vi "JSONRPC Server.vi"(6 "LabVIEW Web Service":refnum<class "Web Service.lvclass">) -> ()   [LabVIEW 2016]
uses:
  <vilib>/wsapi/Web Service.lvclass
  <vilib>/NI/NI JSONRPC Server Framework/Classes/Request/Request.lvclass/Request.ctl
  <vilib>/NI/NI JSONRPC Server Framework/Classes/Request/request.Read method.vi
  <vilib>/NI/NI JSONRPC Server Framework/Classes/Request/request.Read params.vi
  <vilib>/NI/NI JSONRPC Server Framework/Classes/params/params.To JSON Tree.vi
  <vilib>/NI/JSON Support for LabVIEW/JSON Value/New JSON Value/New JSON (String).vi
  <vilib>/NI/NI JSONRPC Server Framework/Classes/Server/Add Response (Method Not Found from Request).vi
  <vilib>/NI/NI JSONRPC Server Framework/Classes/Server/Add Response (Result from Request).vi
  <vilib>/NI/NI JSONRPC Server Framework/Classes/Server/Add Response (Server Error from Request).vi
  <vilib>/NI/JSON Support for LabVIEW/JSON Value/JSON Value.lvclass
  <vilib>/NI/NI JSONRPC Server Framework/Classes/Server/JSONRPC Server.lvclass
  <vilib>/NI/NI JSONRPC Server Framework/Classes/Request/Request.lvclass
panel:
  # "Use the web service input terminal to call the VIs on the Service subpalette of the Web Services palette. Do not remove it from the connector pane unless you don't need access to the palette."
  # "Any additional terminals added to the connector pane of a startup VI will be ignored."
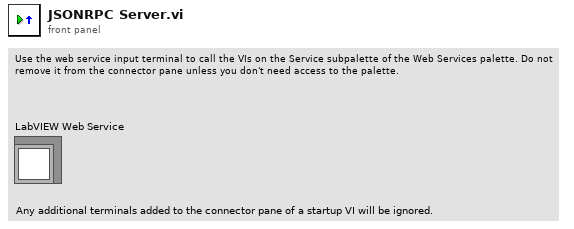
[diagram p1: front panel]
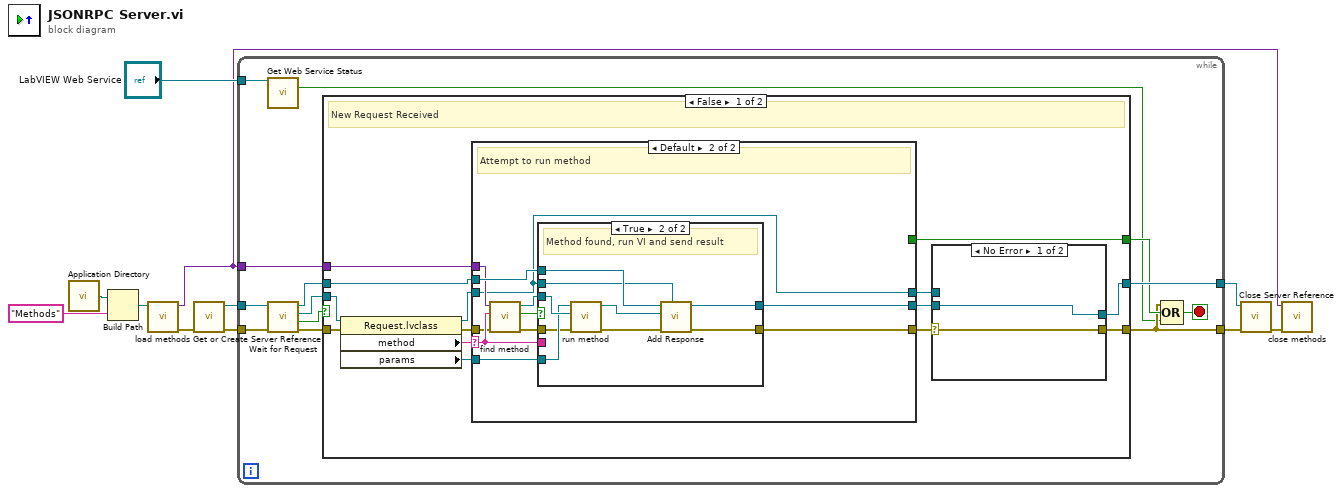
[diagram p0: block diagram]
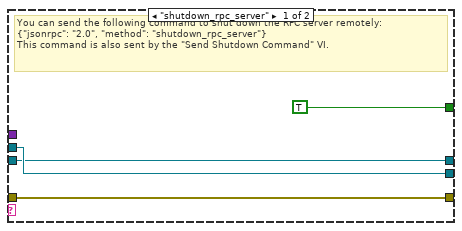
[diagram p2: hidden frame]
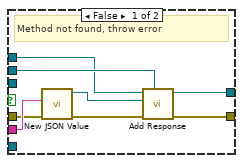
[diagram p3: hidden frame]
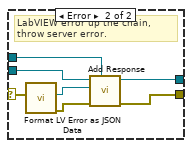
[diagram p4: hidden frame]
diagram:
  n1 = call <vilib>:"Application Directory.vi"() -> ("Application Directory"=w6:path)
  n2 = Build Path(base path=w6, name or relative path="Methods") -> (appended path=w3:path)
  n3 = call "load methods.vi"("Folder Path"=w3) -> ("error out"=w4:errorcluster, "Variant"=w2:variant)  [unwired: 9 in]
  n4 = call <vilib>:"Get or Create Server Reference.vi"("error in (no error)"=w4) -> ("error out"=w10:errorcluster, "Server Out"=w11:refnum<class "JSONRPC Server.lvclass">)  [unwired: 9 in]
  n5 = while {
    tunnel: w11 -> [w24]
    tunnel: w10 -> [w20]
    tunnel: [w16] -> w8
    tunnel: [w18] -> w9
    tunnel: "LabVIEW Web Service" -> [w14]
    tunnel: w2 -> [w12]
    stop <- w15 stop-if-true
    n6 = call <vilib>:"Get Web Service Status.vi"("LabVIEW Web Service"=w14) -> ("service stopping?"=w13:bool)  [unwired: 12 in, 2 out]
    n7 = call <vilib>:"Wait for Request.vi"("error in (no error)"=w20, "Server in"=w24) -> ("error out"=w19:errorcluster, "timed out?"=w21:bool, "Request"=w22:refnum<class "Request.lvclass">, "Server out"=w23:refnum<class "JSONRPC Server.lvclass">)  [unwired: 6 in]
    n8 = case shown="False" w21 {
      tunnel: w23 -> [w29 w80]
      tunnel: w22 -> [w38 _]
      tunnel: w19 -> [w35 w81]
      tunnel: [w30 w81] -> w16
      tunnel: [w33 _] -> w17
      tunnel: [w25 w80] -> w18
      tunnel: w12 -> [w32 _]
      frame False {
        # "New Request Received"
        n9 = property class="Request.lvclass"(reference=w38, error in=w35) -> (reference out=w28:refnum<class "Request.lvclass">, error out=w34:errorcluster, "method"=w37:string, "params"=w36:refnum<class "JSON Value.lvclass">)
        n10 = case shown="Default" w37 {
          selector: w37 -> [_ w49]
          tunnel: w36 -> [_ w50]
          tunnel: w34 -> [w41 w48]
          tunnel: [w41 w52] -> w31
          tunnel: [TRUE _] -> w33
          tunnel: w29 -> [w40 w53]
          tunnel: [w40 w51] -> w26
          tunnel: w28 -> [w39 w43]
          tunnel: w32 -> [_ w44]
          tunnel: [w39 w43] -> w27
          frame "shutdown_rpc_server" {
            # "You can send the following command to shut down the RPC server remotely:\n{\"jsonrpc\": \"2.0\", \"method\": \"shutdown_rpc_server\"}\nThis command is also sent by the \"Send Shutdown Command\" VI."
          }
          frame Default {
            # "Attempt to run method"
            n11 = call "find method.vi"("error in (no error)"=w48, "String"=w49, "Variant"=w44) -> ("error out"=w45:errorcluster, "Boolean"=w46:bool, "VI out"=w47:refnum<vi>)  [unwired: 6 in]
            n12 = case shown="True" w46 {
              tunnel: w53 -> [w60 w70]
              tunnel: w43 -> [w61 w69]
              tunnel: [w58 w68] -> w52
              tunnel: [w59 w67] -> w51
              tunnel: w47 -> [_ w66]
              tunnel: w50 -> [_ w65]
              tunnel: w49 -> [w57 _]
              tunnel: w45 -> [w54 w63]
              frame False {
                # "Method not found, throw error"
                n13 = call-poly <vilib>:"New JSON Value.vi"("error in (no error)"=w54, "value"=w57) -> ("error out"=w55:errorcluster, "JSON Value out"=w56:refnum<class "JSON Value.lvclass">)  [unwired: 8 in]
                n14 = call-poly <vilib>:"Add Response.vi"("Request"=w61, "error in (no error)"=w55, "data"=w56, "Server in"=w60) -> ("error out"=w58:errorcluster, "Server out"=w59:refnum<class "JSONRPC Server.lvclass">)  [unwired: 5 in, 1 out]
              }
              frame True {
                # "Method found, run VI and send result"
                n15 = call "run method.vi"("error in (no error)"=w63, "VI in"=w66, "JSON Value in"=w65) -> ("error out"=w62:errorcluster, "JSON Value out"=w64:refnum<class "JSON Value.lvclass">)  [unwired: 7 in]
                n16 = call-poly <vilib>:"Add Response.vi"("Request"=w69, "error in (no error)"=w62, "JSON Value in"=w64, "Server in"=w70) -> ("error out"=w68:errorcluster, "Server out"=w67:refnum<class "JSONRPC Server.lvclass">)  [unwired: 5 in, 1 out]
              }
            }
          }
        }
        n17 = case shown="No Error" w31 {
          selector: w31 -> [w71 w77]
          tunnel: [w71 w76] -> w30
          tunnel: w27 -> [_ w75]
          tunnel: w26 -> [w72 w74]
          tunnel: [w72 w73] -> w25
          frame No Error {
          }
          frame Error {
            # "LabVIEW error up the chain, throw server error."
            n18 = call <vilib>:"Format LV Error as JSON Data.vi"("error in"=w77) -> ("error out"=w78:errorcluster, "Error Value out"=w79:refnum<class "JSON Value.lvclass">)  [unwired: 9 in]
            n19 = call-poly <vilib>:"Add Response.vi"("Request"=w75, "error in (no error)"=w78, "data"=w79, "Server in"=w74) -> ("error out"=w76:errorcluster, "Server out"=w73:refnum<class "JSONRPC Server.lvclass">)  [unwired: 5 in, 1 out]
          }
        }
      }
      frame True {
        # "Timeout while waiting for new Requests"
      }
    }
    n20 = Compound Arithmetic op=OR(w16, w17, w13) -> (w15:bool)
  }
  n21 = call <vilib>:"Close Server Reference.vi"("error in (no error)"=w8, "Server in"=w9) -> ("error out"=w1:errorcluster)  [unwired: 9 in]
  n22 = call "close methods.vi"("error in (no error)"=w1, "Variant"=w2) -> ()  [unwired: 9 in, 1 out]
